vi "REQ Update Sample Rate.vi"(8 "error in":errorcluster, 10 "Timing Parameter":T1={"rate"=1000.0, "samples per channel"=1000, "sample mode"=10123} {"sample mode" items=["Finite Samples"=10178, "Continuous Samples"=10123, "Hardware Timed Single Point"=12522]; "rate" format="%0.2f"}) -> (0 "error out":errorcluster)   [LabVIEW 2021, in "DAQ Hardware.lvlib"]
doc: "_____\nCreated using DQMH Event Scripter 6.1.0.128."
uses:
  DAQ Hardware.lvlib
  Timing AI DAQ Setting.ctl
  REQ Update Sample Rate Argument--cluster.ctl
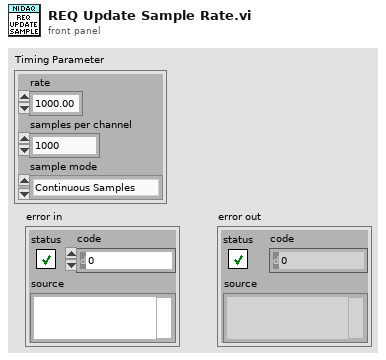
[diagram p1: front panel]
types:
  T1 = typedef "DAQ Hardware.lvlib/Timing AI DAQ Setting.ctl" = cluster{"rate":dbl, "samples per channel":i32, "sample mode":i32}
  T2 = typedef "DAQ Hardware.lvlib/REQ Update Sample Rate Argument--cluster.ctl" = cluster{"Timing Parameter":T1}
  T3 = typedef "DAQ Hardware.lvlib/Request Events--cluster.ctl" = cluster{"Stop Module":refnum<user-event>, "Show Panel":refnum<user-event>, "Hide Panel":refnum<user-event>, "Get Module Execution Status":refnum<user-event>, "Show Diagram":refnum<user-event>, "REQ Initialize AI":refnum<user-event>, "REQ Initialize AO":refnum<user-event>, "REQ Initialize DI":refnum<user-event>, "REQ Initialize DO":refnum<user-event>, "REQ Write DO":refnum<user-event>, "REQ Acquire AI":refnum<user-event>, "REQ Close Ref":refnum<user-event>, "REQ Write AO":refnum<user-event>, "REQ Update Sample Rate":refnum<user-event>, "REQ Acquire DI":refnum<user-event>, "REQ Wakeup_Helper_loop_AI":refnum<user-event>, "REQ Retry AI":refnum<user-event>, "REQ Wakeup_helper_loop_DI":refnum<user-event>, "REQ Retry DI":refnum<user-event>}
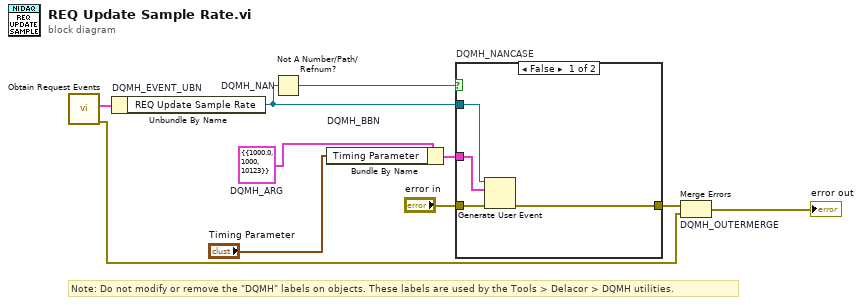
[diagram p0: block diagram]
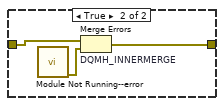
[diagram p2: hidden frame]
diagram:
  w4 = T2 {"Timing Parameter"={"rate"=1000.0, "samples per channel"=1000, "sample mode"=10123}}  # DQMH_ARG
  # "Note: Do not modify or remove the \"DQMH\" labels on objects. These labels are used by the Tools > Delacor > DQMH utilities."
  n1 = call "Obtain Request Events.vi"() -> ("error out"=w2:errorcluster, "DAQ Hardware Request Events"=w1:T3)  [unwired: 10 in]
  n2 = Unbundle By Name "DQMH_EVENT_UBN"(w1) -> ("REQ Update Sample Rate"=w6:refnum<user-event>)
  n3 = Not A Number/Path/Refnum? "DQMH_NAN"(number/path/refnum=w6) -> (NaN/Path/Refnum?=w7:bool)
  n4 = Bundle By Name "DQMH_BBN"(cluster=w4, "Timing Parameter"="Timing Parameter") -> (w8:T2)
  n5 = case "DQMH_NANCASE" shown="False" w7 {
    tunnel: "error in" -> [w14 w17]
    tunnel: [w13 w16] -> w5
    tunnel: w6 -> [w12 _]
    tunnel: w8 -> [w11 _]
    frame False {
      n6 = Generate User Event(user event=w12, event data cluster=w11, error in=w14) -> (error out=w13:errorcluster)  [unwired: 1 in, 1 out]
    }
    frame True {
      n7 = call "Module Not Running--error.vi"() -> ("error out"=w15:errorcluster)  [unwired: 11 in]
      n8 = Merge Errors "DQMH_INNERMERGE"(w17, w15) -> (w16:errorcluster)
    }
  }
  n9 = Merge Errors "DQMH_OUTERMERGE"(w5, w2) -> (→"error out":errorcluster)
